vi "TEMPDo.vi"(8 "error in (no error)":errorcluster, 10 "Actor in":refnum<class "Actor.lvclass">, 11 "DNL_Message Template":refnum<class "Message.lvclass">) -> (0 "error out":errorcluster, 2 "Actor out":refnum<class "Actor.lvclass">)   [LabVIEW 2016, in "Message Template.lvclass"]
doc: "This VI delivers the message to the actor by calling the appropriate method(s) on the actor."
uses:
  Message Template.lvclass
  <vilib>/ActorFramework/Actor/Actor.lvclass
  <vilib>/ActorFramework/Message/Message.lvclass
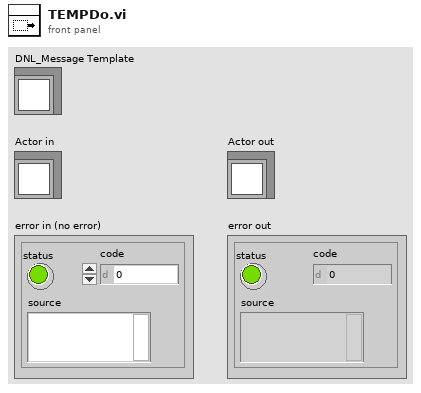
[diagram p1: front panel]
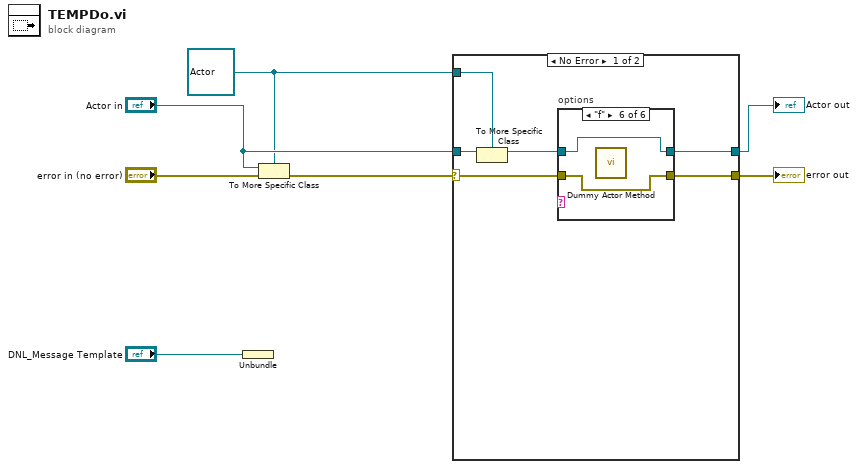
[diagram p0: block diagram]
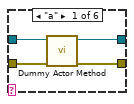
[diagram p2: hidden frame]
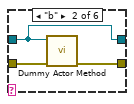
[diagram p3: hidden frame]
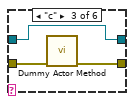
[diagram p4: hidden frame]
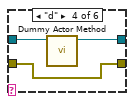
[diagram p5: hidden frame]
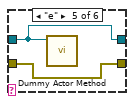
[diagram p6: hidden frame]
diagram:
  w2 = refnum<class "Actor.lvclass"> refnum ("Actor in")
  n1 = Unbundle ("Main-Unbundle")("DNL_Message Template") -> ()  [unwired: 1 out]
  n2 = To More Specific Class(target class=w2, reference="Actor in", error in="error in (no error)") -> (error out=w6:errorcluster)  [unwired: 1 out]
  n3 = case shown="No Error" w6 {
    selector: w6 -> [w11 w32]
    tunnel: [w13 w32] -> w5
    tunnel: [w12 w31] -> w4
    tunnel: "Actor in" -> [w10 w31]
    tunnel: w2 -> [w9 _]
    frame No Error {
      n4 = To More Specific Class(target class=w9, reference=w10) -> (specific class reference=w8:refnum<class "Actor.lvclass">)  [unwired: 1 in, 1 out]
      n5 = case "options" shown="\"f\"" {
        selector: _ -> [_ _ _ _ _ _]
        tunnel: [w17 w20 w23 w26 w27 w29] -> w13
        tunnel: [w16 w18 w21 w24 w28 w30] -> w12
        tunnel: w11 -> [w15 w19 w22 w26 w27 w29]
        tunnel: w8 -> [w14 w18 w21 w25 w28 w30]
        frame "a" {
          n6 = call "Dummy Actor Method.vi"("error in (no error)"=w15, "Actor in"=w14) -> ("error out"=w17:errorcluster, "Actor out"=w16:refnum<class "Actor.lvclass">)  [unwired: 8 in]
        }
        frame "b" {
          n7 = call "Dummy Actor Method.vi"("error in (no error)"=w19, "Actor in"=w18) -> ("error out"=w20:errorcluster)  [unwired: 8 in, 1 out]
        }
        frame "c" {
          n8 = call "Dummy Actor Method.vi"("error in (no error)"=w22) -> ("error out"=w23:errorcluster)  [unwired: 9 in, 1 out]
        }
        frame "d" {
          n9 = call "Dummy Actor Method.vi"("Actor in"=w25) -> ("Actor out"=w24:refnum<class "Actor.lvclass">)  [unwired: 9 in, 1 out]
        }
        frame "e" {
          n10 = call "Dummy Actor Method.vi"("Actor in"=w28) -> ()  [unwired: 9 in, 2 out]
        }
        frame "f" {
          n11 = call "Dummy Actor Method.vi"() -> ()  [unwired: 10 in, 2 out]
        }
      }
    }
    frame Error {
    }
  }
  "error out" <- w5
  "Actor out" <- w4
